vi "Misure pre misura resistomat.vi"(10 "Misure":T1, 11 "Pre resistomat":T1) -> (3 "Misure out":T1)   [LabVIEW 2019]
uses:
  TypeDef/MISURE NM.ctl
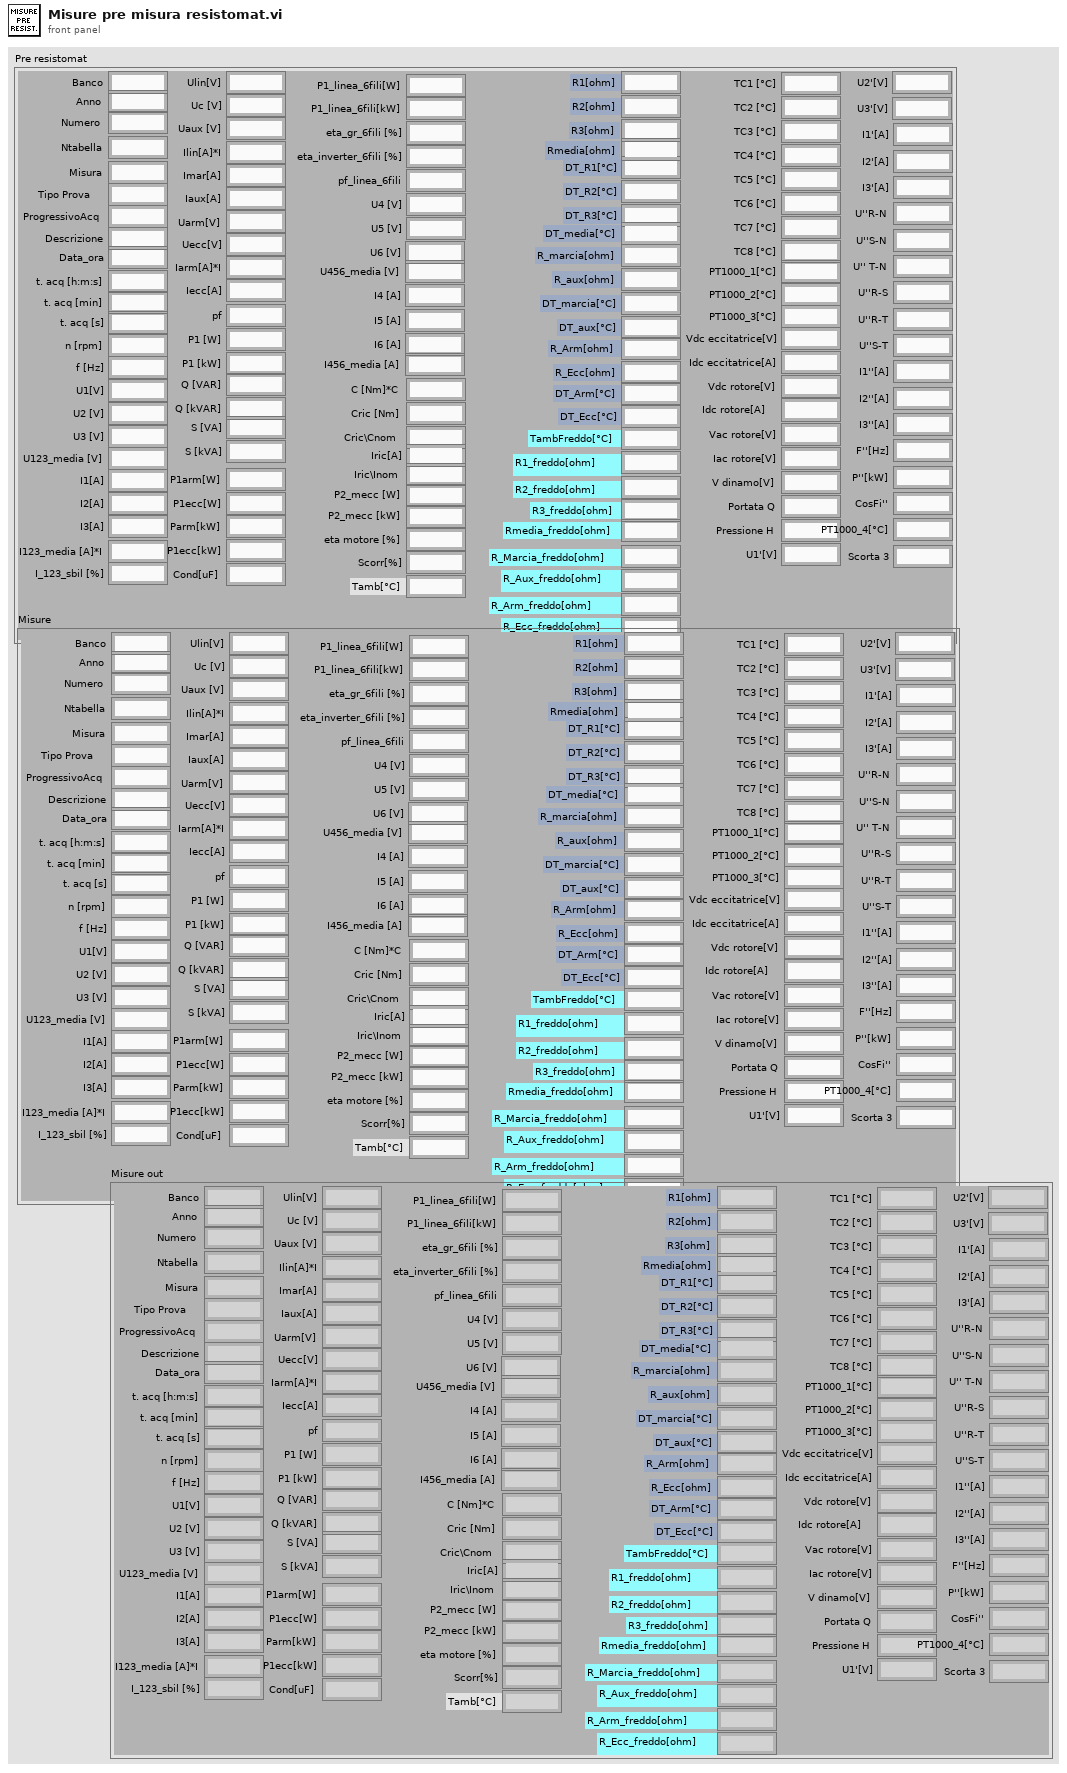
[diagram p1: front panel]
types:
  T1 = typedef "MISURE NM.ctl" = cluster{"Banco":string, "Anno":string, "Numero":string, "Ntabella":string, "Misura":string, "Tipo Prova":string, "ProgressivoAcq":string, "Descrizione":string, "Data_ora":string, "t. acq [h:m:s]":string, "t. acq [min]":string, "t. acq [s]":string, "n [rpm]":string, "f [Hz]":string, "U1[V]":string, "U2 [V]":string, "U3 [V]":string, "U123_media [V]":string, "I1[A]":string, "I2[A]":string, "I3[A]":string, "I123_media [A]*I":string, "I_123_sbil [%]":string, "Ulin[V]":string, "Uc [V]":string, "Uaux [V]":string, "Ilin[A]*I":string, "Imar[A]":string, "Iaux[A]":string, "Uarm[V]":string, "Uecc[V]":string, "Iarm[A]*I":string, "Iecc[A]":string, "pf":string, "P1 [W]":string, "P1 [kW]":string, "Q [VAR]":string, "Q [kVAR]":string, "S [VA]":string, "S [kVA]":string, "P1arm[W]":string, "P1ecc[W]":string, "Parm[kW]":string, "P1ecc[kW]":string, "Cond[uF]":string, "P1_linea_6fili[W]":string, "P1_linea_6fili[kW]":string, "eta_gr_6fili [%]":string, "eta_inverter_6fili [%]":string, "pf_linea_6fili":string, "U4 [V]":string, "U5 [V]":string, "U6 [V]":string, "U456_media [V]":string, "I4 [A]":string, "I5 [A]":string, "I6 [A]":string, "I456_media [A]":string, "C [Nm]*C":string, "Cric [Nm]":string, "Cric\\Cnom":string, "Iric[A]":string, "Iric\\Inom":string, "P2_mecc [W]":string, "P2_mecc [kW]":string, "eta motore [%]":string, "Scorr[%]":string, "Tamb[°C]":string, "R1[ohm]":string, "R2[ohm]":string, "R3[ohm]":string, "Rmedia[ohm]":string, "DT_R1[°C]":string, "DT_R2[°C]":string, "DT_R3[°C]":string, "DT_media[°C]":string, "R_marcia[ohm]":string, "R_aux[ohm]":string, "DT_marcia[°C]":string, "DT_aux[°C]":string, "R_Arm[ohm]":string, "R_Ecc[ohm]":string, "DT_Arm[°C]":string, "DT_Ecc[°C]":string, "TambFreddo[°C]":string, "R1_freddo[ohm]":string, "R2_freddo[ohm]":string, "R3_freddo[ohm]":string, "Rmedia_freddo[ohm]":string, "R_Marcia_freddo[ohm]":string, "R_Aux_freddo[ohm]":string, "R_Arm_freddo[ohm]":string, "R_Ecc_freddo[ohm]":string, "TC1 [°C]":string, "TC2 [°C]":string, "TC3 [°C]":string, "TC4 [°C]":string, "TC5 [°C]":string, "TC6 [°C]":string, "TC7 [°C]":string, "TC8 [°C]":string, "PT1000_1[°C]":string, "PT1000_2[°C]":string, "PT1000_3[°C]":string, "Vdc eccitatrice[V]":string, "Idc eccitatrice[A]":string, "Vdc rotore[V]":string, "Idc rotore[A]":string, "Vac rotore[V]":string, "Iac rotore[V]":string, "V dinamo[V]":string, "Portata Q":string, "Pressione H":string, "U1'[V]":string, "U2'[V]":string, "U3'[V]":string, "I1'[A]":string, "I2'[A]":string, "I3'[A]":string, "U''R-N":string, "U''S-N":string, "U'' T-N":string, "U''R-S":string, "U''R-T":string, "U''S-T":string, "I1''[A]":string, "I2''[A]":string, "I3''[A]":string, "F''[Hz]":string, "P''[kW]":string, "CosFi''":string, "PT1000_4[°C]":string, "Scorta 3":string}
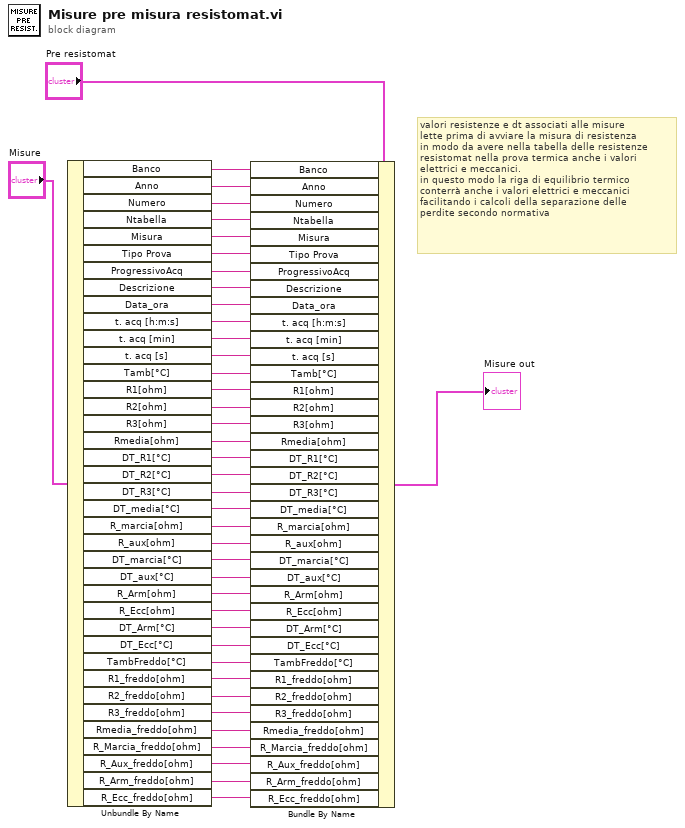
[diagram p0: block diagram]
diagram:
  # "valori resistenze e dt associati alle misure \nlette prima di avviare la misura di resistenza\nin modo da avere nella tabella delle resistenze\nresistomat nella prova termica anche i valori\nelettrici e meccanici.\nin questo modo la riga di equilibrio termico\nconterrà anche i valori elettrici e meccanici\nfacilitando i calcoli della separazione delle\nperdite secondo normativa"
  n1 = Unbundle By Name("Misure") -> ("Banco"=w39:string, "Anno"=w38:string, "Numero"=w37:string, "Ntabella"=w36:string, "Misura"=w35:string, "Tipo Prova"=w34:string, "ProgressivoAcq"=w33:string, "Descrizione"=w32:string, "Data_ora"=w31:string, "t. acq [h:m:s]"=w30:string, "t. acq [min]"=w29:string, "t. acq [s]"=w28:string, "Tamb[°C]"=w27:string, "R1[ohm]"=w26:string, "R2[ohm]"=w25:string, "R3[ohm]"=w24:string, "Rmedia[ohm]"=w3:string, "DT_R1[°C]"=w4:string, "DT_R2[°C]"=w23:string, "DT_R3[°C]"=w22:string, "DT_media[°C]"=w6:string, "R_marcia[ohm]"=w5:string, "R_aux[ohm]"=w21:string, "DT_marcia[°C]"=w20:string, "DT_aux[°C]"=w19:string, "R_Arm[ohm]"=w18:string, "R_Ecc[ohm]"=w17:string, "DT_Arm[°C]"=w16:string, "DT_Ecc[°C]"=w15:string, "TambFreddo[°C]"=w13:string, "R1_freddo[ohm]"=w12:string, "R2_freddo[ohm]"=w11:string, "R3_freddo[ohm]"=w10:string, "Rmedia_freddo[ohm]"=w1:string, "R_Marcia_freddo[ohm]"=w2:string, "R_Aux_freddo[ohm]"=w9:string, "R_Arm_freddo[ohm]"=w8:string, "R_Ecc_freddo[ohm]"=w7:string)
  n2 = Bundle By Name(cluster="Pre resistomat", "Banco"=w39, "Anno"=w38, "Numero"=w37, "Ntabella"=w36, "Misura"=w35, "Tipo Prova"=w34, "ProgressivoAcq"=w33, "Descrizione"=w32, "Data_ora"=w31, "t. acq [h:m:s]"=w30, "t. acq [min]"=w29, "t. acq [s]"=w28, "Tamb[°C]"=w27, "R1[ohm]"=w26, "R2[ohm]"=w25, "R3[ohm]"=w24, "Rmedia[ohm]"=w3, "DT_R1[°C]"=w4, "DT_R2[°C]"=w23, "DT_R3[°C]"=w22, "DT_media[°C]"=w6, "R_marcia[ohm]"=w5, "R_aux[ohm]"=w21, "DT_marcia[°C]"=w20, "DT_aux[°C]"=w19, "R_Arm[ohm]"=w18, "R_Ecc[ohm]"=w17, "DT_Arm[°C]"=w16, "DT_Ecc[°C]"=w15, "TambFreddo[°C]"=w13, "R1_freddo[ohm]"=w12, "R2_freddo[ohm]"=w11, "R3_freddo[ohm]"=w10, "Rmedia_freddo[ohm]"=w1, "R_Marcia_freddo[ohm]"=w2, "R_Aux_freddo[ohm]"=w9, "R_Arm_freddo[ohm]"=w8, "R_Ecc_freddo[ohm]"=w7) -> (→"Misure out":T1)
